vi "SI8_Parsing_data.vi"(11 "IN":string="#GHGNUMPSGGGLMKIJKPIIKGRHNP") -> (3 "OUT":string)   [LabVIEW 2018]
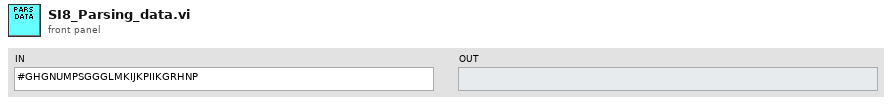
[diagram p1: front panel]
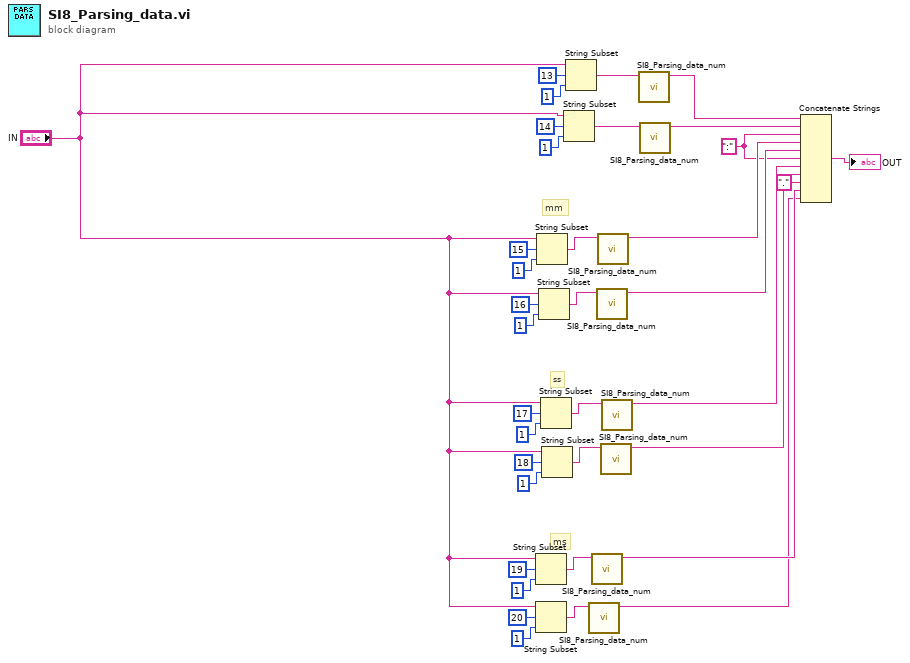
[diagram p0: block diagram]
diagram:
  w16 = ":" ("string")
  # "ms"
  # "ss"
  # "mm"
  n1 = String Subset(string="IN", offset (0)=19, length (rest)=1 ("length (rest)")) -> (substring=w20:string)
  n2 = String Subset(string="IN", offset (0)=20, length (rest)=1 ("length (rest)")) -> (substring=w19:string)
  n3 = String Subset(string="IN", offset (0)=15, length (rest)=1 ("length (rest)")) -> (substring=w24:string)
  n4 = String Subset(string="IN", offset (0)=16, length (rest)=1 ("length (rest)")) -> (substring=w23:string)
  n5 = String Subset(string="IN", offset (0)=17, length (rest)=1 ("length (rest)")) -> (substring=w22:string)
  n6 = String Subset(string="IN", offset (0)=18, length (rest)=1 ("length (rest)")) -> (substring=w21:string)
  n7 = String Subset(string="IN", offset (0)=14, length (rest)=1 ("length (rest)")) -> (substring=w4:string)
  n8 = String Subset(string="IN", offset (0)=13, length (rest)=1 ("length (rest)")) -> (substring=w3:string)
  n9 = call "SI8_Parsing_data_num.vi"("Input"=w19) -> ("Choice"=w11:string)  [unwired: 10 in]
  n10 = call "SI8_Parsing_data_num.vi"("Input"=w20) -> ("Choice"=w12:string)  [unwired: 10 in]
  n11 = call "SI8_Parsing_data_num.vi"("Input"=w23) -> ("Choice"=w17:string)  [unwired: 10 in]
  n12 = call "SI8_Parsing_data_num.vi"("Input"=w24) -> ("Choice"=w18:string)  [unwired: 10 in]
  n13 = call "SI8_Parsing_data_num.vi"("Input"=w21) -> ("Choice"=w14:string)  [unwired: 10 in]
  n14 = call "SI8_Parsing_data_num.vi"("Input"=w22) -> ("Choice"=w15:string)  [unwired: 10 in]
  n15 = call "SI8_Parsing_data_num.vi"("Input"=w3) -> ("Choice"=w1:string)  [unwired: 10 in]
  n16 = call "SI8_Parsing_data_num.vi"("Input"=w4) -> ("Choice"=w2:string)  [unwired: 10 in]
  n17 = Concatenate Strings(w1, w2, w16, w18, w17, w16, w15, w14, "." ("string"), w12, w11) -> (→"OUT":string)
